vi "WriteFirmwareInfoUSB.vi"(8 "error in (no error)":errorcluster, 11 "path":path) -> (0 "error out":errorcluster)   [LabVIEW 2017, in "USBDrive.lvlib"]
uses:
  <vilib>/addons/InsightCM/Devices/Shared/Common/USBDrive/USBDrive.lvlib
  <vilib>/addons/SystemInfoProcess/SystemInfoProcess.lvlib
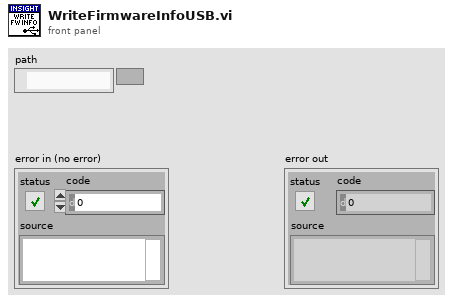
[diagram p1: front panel]
types:
  T1 = typedef "PointValueMap.lvlib/PointMap.ctl" = refnum<data-value>
  T2 = typedef "SystemInfoProcess.lvlib/ImageMetadata.ctl" = cluster{"Title":string, "Description":string, "ID":string, "Version":string}
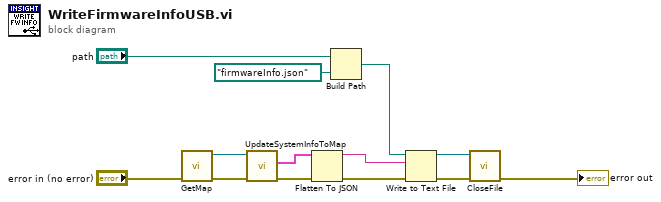
[diagram p0: block diagram]
diagram:
  n1 = call <vilib>:"GetMap.vi"("error in (no error)"="error in (no error)") -> ("error out"=w9:errorcluster, "SystemInfoMap"=w11:T1)  [unwired: 9 in]
  n2 = call <vilib>:"UpdateSystemInfoToMap.vi"("error in (no error)"=w9, "map in"=w11) -> ("error out"=w8:errorcluster, "system info"=w10:T2)  [unwired: 5 in, 3 out]
  n3 = Flatten To JSON(anything=w10, error in (no error)=w8) -> (JSON string=w6:string, 11:w7:errorcluster)  [unwired: 1 in]
  n4 = Build Path(base path="path", name or relative path=path "firmwareInfo.json" ("dup path")) -> (appended path=w13:path)
  n5 = Write to Text File(file (use dialog)=w13, text=w6, error in=w7) -> (refnum out=w3:refnum<file>, error out=w2:errorcluster)  [unwired: 1 in, 1 out]
  n6 = call <vilib>:"CloseFile.vi"("error in (no error)"=w2, "file reference"=w3) -> ("error out"=→"error out":errorcluster)  [unwired: 9 in]
